vi "Shared Variable Selection RTM.vi"(8 "error in (no error)":errorcluster, 11 "Node Ptr":u64 format="%.0x") -> (0 "error out":errorcluster)   [LabVIEW 2012, in "Shared Variable Custom Device.lvlib"]
uses:
  Shared Variable Custom Device.lvlib
  Shared/Shared Variable GUID Lookup.vi
panel:
  in  "Previous Button":bool
  in  "Cancel Button":bool
  in  "OK Button":bool
  in  "Next Button":bool
  in  "VeriStand Tree":string[](tree)
  in  "Shared Variable Tree":string[](tree)
  in  "Tag":string
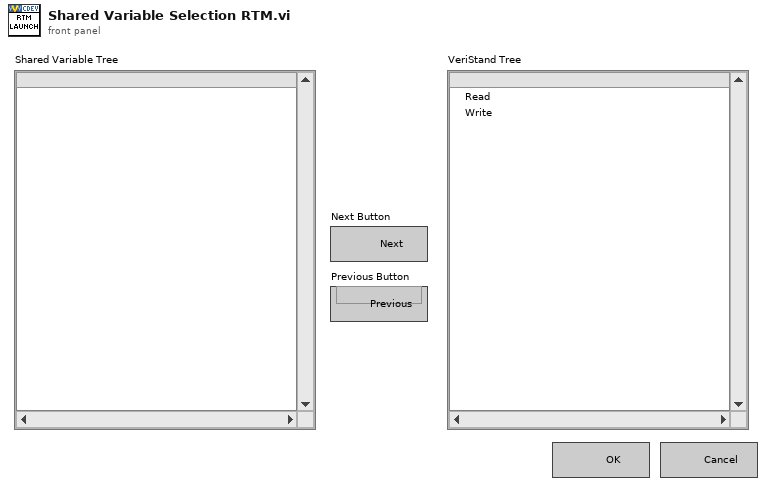
[diagram p1: front panel]
types:
  T1 = typedef "Custom Device API.lvlib/Custom Device Item Ref.ctl" = u64
  T2 = typedef "Shared Variable Custom Device.lvlib/Existing Channel Data.ctl" = cluster{"Sh Var URL":string[], "VS Name":string[], "Sh Var Name":string[], "Data Type":T3[]}
  T3 = typedef "VariantType.lvlib/Type.ctl" = enum8{"Invalid Type", "Void", "I8", "I16", "I32", "I64", "U8", "U16", "U32", "U64", "Single Float", "Double Float", "Extended Float", "Single Complex", "Double Complex", "Extended Complex", "Enum U8", "Enum U16", "Enum U32", "Enum U64", "Single Float With Unit", "Double Float With Unit", "Extended Float With Unit", "Single Complex with Unit", "Double Complex with Unit", "Extended Complex with Unit", "Boolean", "String", "Path", "Picture", "Tag", "Array", "Cluster", "Variant", "LV Variant", "Waveform", "Timestamp", "Digital Waveform", "Digital Data", "ExpressData", "Refnum", "External Data", "VI", "Poly VI", "LabVIEW Class Instance", "Fixed Point"}
  T4 = typedef "Shared Variable Custom Device.lvlib/Tree Data.ctl" = cluster{"Child Tag":string, "Parent Tag":string, "VS Name":string, "Sh Var Name":string, "Sh Var URL":string, "Data Type":T3, "Symbol":i32}
  T5 = typedef "Shared Variable Custom Device.lvlib/List Cluster.ctl" = cluster{"Shared Variable List":T4[], "Read List":T4[], "Write List":T4[]}
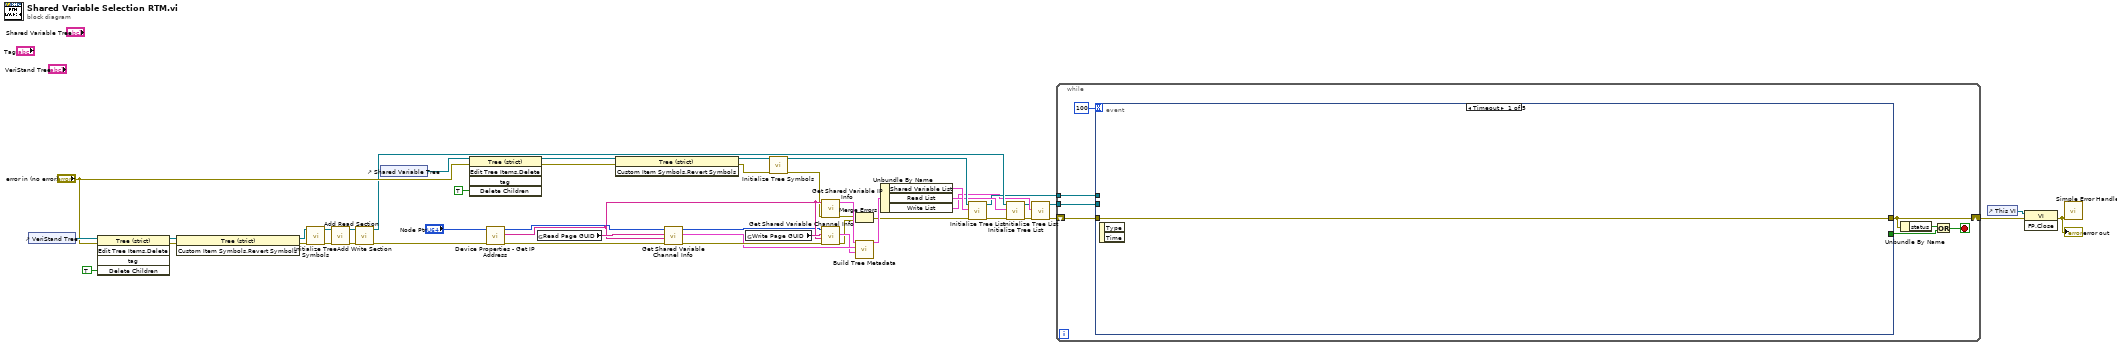
[diagram p0: block diagram]
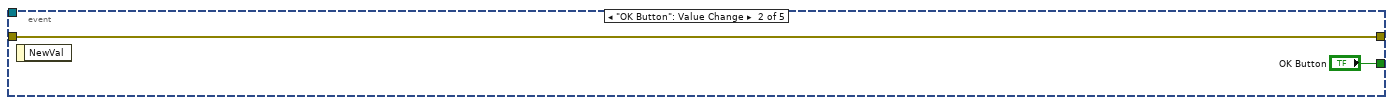
[diagram p2: hidden frame]
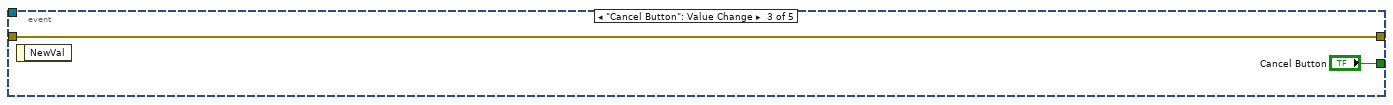
[diagram p3: hidden frame]
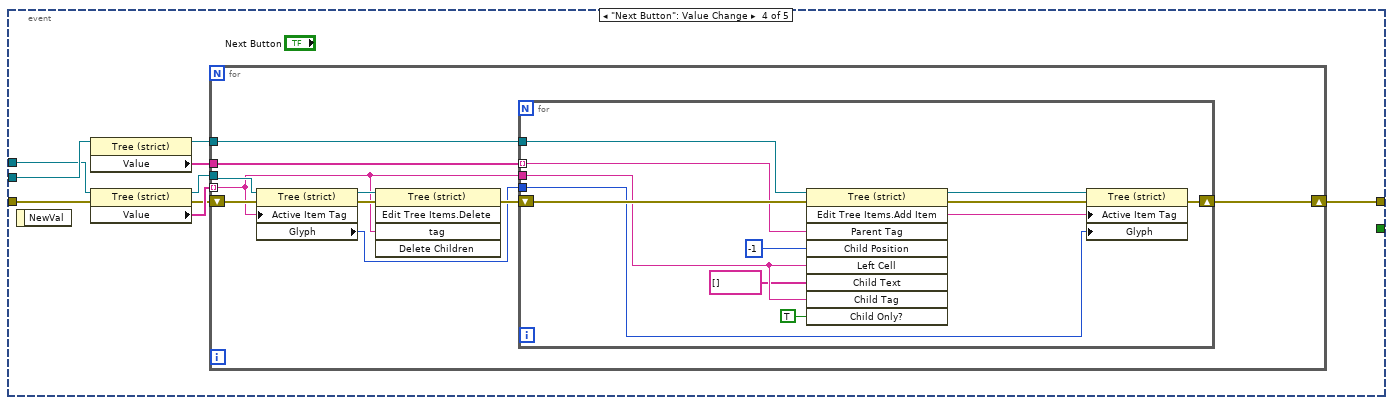
[diagram p4: hidden frame]
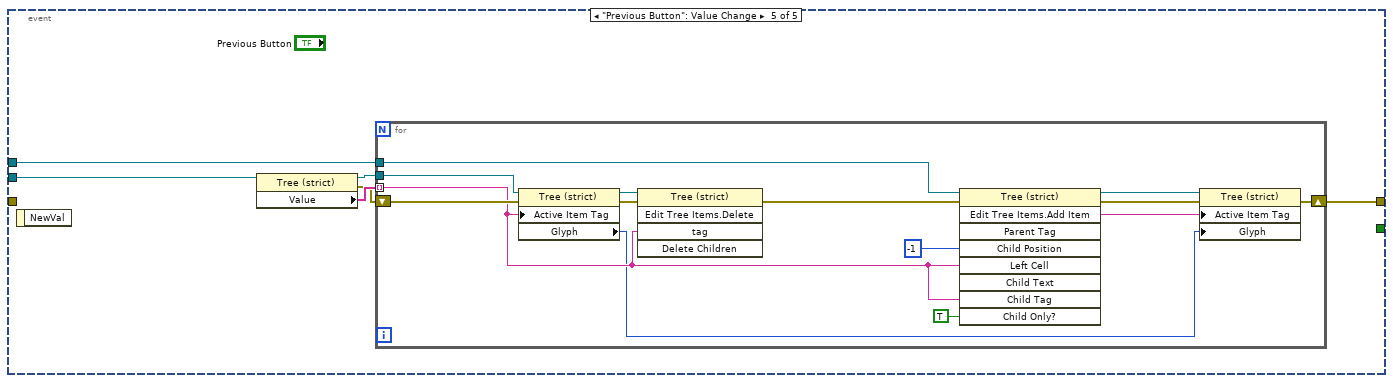
[diagram p5: hidden frame]
diagram:
  n1 = control-ref of="VeriStand Tree"() -> (w34:refnum<vi>)
  n2 = invoke class="Tree (strict)" method="Edit Tree Items.Delete"(reference=w34, error in="error in (no error)", "Delete Children"=TRUE ("Delete Children?")) -> (reference out=w36:refnum<vi>, error out=w37:errorcluster)  [unwired: 2 in, 3 out]
  n3 = invoke class="Tree (strict)" method="Custom Item Symbols.Revert Symbols"(reference=w36, error in=w37) -> (reference out=w28:refnum<vi>, error out=w32:errorcluster)  [unwired: 1 in, 1 out]
  n4 = call "Initialize Tree Symbols.vi"("error in (no error)"=w32, "TreeControl in"=w28) -> ("error out"=w26:errorcluster, "TreeControl out"=w30:refnum<vi>)  [unwired: 8 in]
  n5 = call "Add Read Section.vi"("error in (no error)"=w26, "TreeControl in"=w30) -> ("error out"=w25:errorcluster, "TreeControl out"=w24:refnum<vi>)  [unwired: 7 in, 1 out]
  n6 = call "Add Write Section.vi"("error in (no error)"=w25, "TreeControl in"=w24) -> ("error out"=w23:errorcluster, "TreeControl out"=w10:refnum<vi>)  [unwired: 7 in, 1 out]
  n7 = control-ref of="Shared Variable Tree"() -> (w48:refnum<vi>)
  n8 = invoke class="Tree (strict)" method="Edit Tree Items.Delete"(reference=w48, error in="error in (no error)", "Delete Children"=TRUE ("Delete Children?")) -> (reference out=w46:refnum<vi>, error out=w45:errorcluster)  [unwired: 2 in, 3 out]
  n9 = call "Device Properties - Get IP Address.vi"("error in (no error)"=w23, "Device Ref in"="Node Ptr") -> ("error out"=w42:errorcluster, "IP Address"=w38:string, "Device Ref out"=w41:T1)  [unwired: 7 in]
  n10 = global read "Shared Variable GUID Lookup.vi" "Read Page GUID"() -> (w40:string)
  n11 = invoke class="Tree (strict)" method="Custom Item Symbols.Revert Symbols"(reference=w46, error in=w45) -> (reference out=w27:refnum<vi>, error out=w44:errorcluster)  [unwired: 1 in, 1 out]
  n12 = call "Get Shared Variable Channel Info.vi"("error in (no error)"=w42, "IP Address"=w38, "Section GUID"=w40, "Device Ref in"=w41) -> ("error out"=w22:errorcluster, "Shared Variable Channel Info"=w17:T2, "Device Ref out"=w29:T1)  [unwired: 5 in]
  n13 = global read "Shared Variable GUID Lookup.vi" "Write Page GUID"() -> (w39:string)
  n14 = call "Initialize Tree Symbols.vi"("error in (no error)"=w44, "TreeControl in"=w27) -> ("error out"=w31:errorcluster, "TreeControl out"=w15:refnum<vi>)  [unwired: 8 in]
  n15 = call "Get Shared Variable IP Info.vi"("error in (no error)"=w31, "IP Address"=w38) -> ("error out"=w2:errorcluster, "Sh Var Data Array"=w18:T4[])  [unwired: 8 in]
  n16 = call "Get Shared Variable Channel Info.vi"("error in (no error)"=w22, "IP Address"=w38, "Section GUID"=w39, "Device Ref in"=w29) -> ("error out"=w3:errorcluster, "Shared Variable Channel Info"=w16:T2)  [unwired: 5 in, 1 out]
  n17 = Merge Errors(w2, w3) -> (w1:errorcluster)
  n18 = call "Build Tree Metadata.vi"("Write Channel Data in"=w16, "Read Channel Data in"=w17, "Sh Var Data Array"=w18) -> ("List Out"=w14:T5)  [unwired: 6 in, 2 out]
  n19 = Unbundle By Name(w14) -> ("Shared Variable List"=w13:T4[], "Read List"=w11:T4[], "Write List"=w8:T4[])
  n20 = call "Initialize Tree List.vi"("error in (no error)"=w1, "List in"=w13, "TreeControl in"=w15) -> ("error out"=w12:errorcluster, "TreeControl out"=w9:refnum<vi>)  [unwired: 7 in]
  n21 = call "Initialize Tree List.vi"("error in (no error)"=w12, "List in"=w11, "TreeControl in"=w10) -> ("error out"=w7:errorcluster, "TreeControl out"=w6:refnum<vi>)  [unwired: 7 in]
  n22 = call "Initialize Tree List.vi"("error in (no error)"=w7, "List in"=w8, "TreeControl in"=w6) -> ("error out"=w4:errorcluster, "TreeControl out"=w5:refnum<vi>)  [unwired: 7 in]
  n23 = while {
    shift-right: [w53] -> w21
    shift-left: w4 -> [w56]
    tunnel: w9 -> [w49]
    tunnel: w5 -> [w50]
    stop <- w54 stop-if-true
    n24 = event shown="[0] Timeout" {
      selector: _ -> [_ _ _ _ _]
      dyn-events: _ -> [_ _ _ _ _]
      timeout: 100 -> [_ _ _ _ _]
      tunnel: w56 -> [w57 w59 w60 w70 _]
      tunnel: [w57 w59 w60 w65 w95] -> w53
      tunnel: [_ "OK Button" "Cancel Button" _ _] -> w51
      tunnel: w50 -> [_ _ _ w63 w94]
      tunnel: w49 -> [_ _ _ w62 w93]
      event Timeout {
        n25 = event-data() -> ()  [unwired: 1 in, 2 out]
      }
      event "OK Button": Value Change {
        n26 = event-data() -> ()  [unwired: 1 in, 1 out]
      }
      event "Cancel Button": Value Change {
        n27 = event-data() -> ()  [unwired: 1 in, 1 out]
      }
      event "Next Button": Value Change {
        n28 = event-data() -> ()  [unwired: 1 in, 1 out]
        n29 = property class="Tree (strict)"(reference=w63) -> (reference out=w66:refnum<vi>, "Value"=w64:string[])  [unwired: 1 in, 1 out]
        n30 = property class="Tree (strict)"(reference=w62, error in=w70) -> (reference out=w68:refnum<vi>, error out=w67:errorcluster, "Value"=w69:string[])
        n31 = for {
          tunnel: w69 -> [w75] mode=indexing
          tunnel: w68 -> [w79]
          shift-right: [w73] -> w65
          shift-left: w67 -> [w78]
          tunnel: w66 -> [w74]
          tunnel: w64 -> [w71]
          n32 = property class="Tree (strict)"(reference=w79, error in=w78, "Active Item Tag"=w75) -> (reference out=w76:refnum<vi>, error out=w77:errorcluster, "Glyph"=w72:i32)
          n33 = invoke class="Tree (strict)" method="Edit Tree Items.Delete"(reference=w76, error in=w77, "tag"=w75) -> (error out=w80:errorcluster)  [unwired: 2 in, 4 out]
          n34 = for {
            tunnel: w75 -> [w91]
            tunnel: w74 -> [w89]
            tunnel: w72 -> [w84]
            tunnel: w71 -> [w83] mode=indexing
            shift-right: [w88] -> w73
            shift-left: w80 -> [w92]
            n35 = invoke class="Tree (strict)" method="Edit Tree Items.Add Item"(reference=w89, error in=w92, "Parent Tag"=w83, "Child Position"=-1, "Left Cell"=w91, "Child Text"=string[] [], "Child Tag"=w91, "Child Only?"=TRUE) -> (reference out=w86:refnum<vi>, error out=w87:errorcluster, "Edit Tree Items:Add Item"=w85:string)  [unwired: 1 in, 6 out]
            n36 = property class="Tree (strict)"(reference=w86, error in=w87, "Active Item Tag"=w85, "Glyph"=w84) -> (error out=w88:errorcluster)  [unwired: 1 out]
          }
        }
      }
      event "Previous Button": Value Change {
        n37 = event-data() -> ()  [unwired: 1 in, 1 out]
        n38 = property class="Tree (strict)"(reference=w94) -> (reference out=w97:refnum<vi>, error out=w96:errorcluster, "Value"=w98:string[])  [unwired: 1 in]
        n39 = for {
          tunnel: w98 -> [w107] mode=indexing
          tunnel: w97 -> [w111]
          shift-right: [w106] -> w95
          shift-left: w96 -> [w110]
          tunnel: w93 -> [w99]
          n40 = property class="Tree (strict)"(reference=w111, error in=w110, "Active Item Tag"=w107) -> (reference out=w108:refnum<vi>, error out=w109:errorcluster, "Glyph"=w105:i32)
          n41 = invoke class="Tree (strict)" method="Edit Tree Items.Delete"(reference=w108, error in=w109, "tag"=w107) -> (error out=w112:errorcluster)  [unwired: 2 in, 4 out]
          n42 = invoke class="Tree (strict)" method="Edit Tree Items.Add Item"(reference=w99, error in=w112, "Child Position"=-1, "Left Cell"=w107, "Child Tag"=w107, "Child Only?"=TRUE) -> (reference out=w102:refnum<vi>, error out=w103:errorcluster, "Edit Tree Items:Add Item"=w101:string)  [unwired: 3 in, 6 out]
          n43 = property class="Tree (strict)"(reference=w102, error in=w103, "Active Item Tag"=w101, "Glyph"=w105) -> (error out=w106:errorcluster)  [unwired: 1 out]
        }
      }
    }
    n44 = Unbundle By Name(w53) -> ("status"=w52:bool)
    n45 = Or(x=w52, y=w51) -> (x .or. y?=w54:bool)
  }
  n46 = control-ref of="This VI"() -> (w19:refnum<vi>)
  n47 = invoke class="VI" method="FP.Close"(reference=w19, error in=w21) -> (error out=w20:errorcluster)  [unwired: 1 in, 2 out]
  "error out" <- w20
  n48 = call <vilib>:"Simple Error Handler.vi"("error in (no error)"=w20) -> ()  [unwired: 4 in, 5 out]
